vi "Drive.vi"(8 "error in":errorcluster) -> (0 "error out":errorcluster)   [LabVIEW 2009, in "Main.lvlib"]
uses:
  Main.lvlib
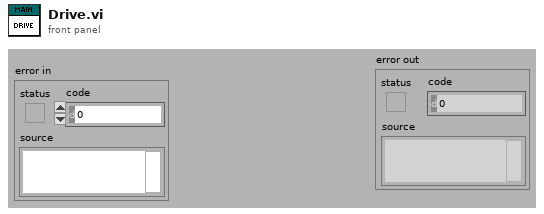
[diagram p1: front panel]
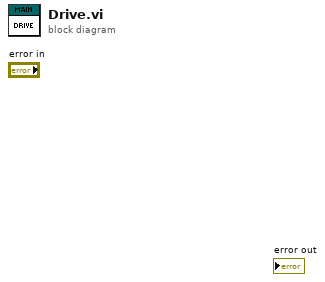
[diagram p0: block diagram]
diagram:
